vi "错误判断-空文件.vi"(8 "错误输入":errorcluster caption="输入簇") -> (0 "无错误输出":errorcluster caption="错误输出", 3 "空文件？":bool)   [LabVIEW 2017]
doc: "1102错误代码：空文件"
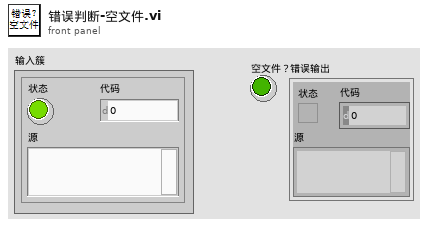
[diagram p1: front panel]
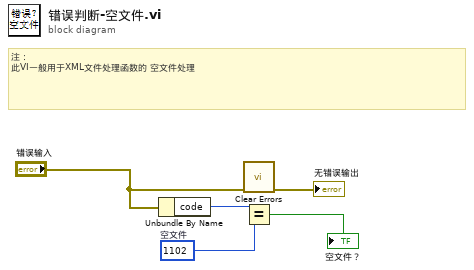
[diagram p0: block diagram]
diagram:
  w4 = 1102  # 空文件
  # "注：\n此VI一般用于XML文件处理函数的 空文件处理"
  n1 = Unbundle By Name("错误输入") -> ("code"=w3:i32)
  n2 = call <vilib>:"Clear Errors.vi"("error in (no error)"="错误输入") -> ("error out"=→"无错误输出":errorcluster)  [unwired: 5 in, 1 out]
  n3 = Equal?(x=w3, y=w4) -> (x = y?=→"空文件？":bool)
